vi "EminemStateToNumb.vi"(11 "Eminim_state":T1) -> (3 "StateNumber":dbl)   [LabVIEW 2023]
uses:
  EminemStatesEnum.ctl
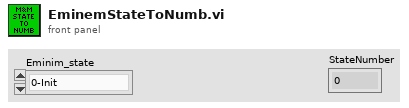
[diagram p1: front panel]
types:
  T1 = typedef "EminemStatesEnum.ctl" = enum16{"0-Init", "1-WaitForCmd", "2-Cancel", "3-ShootStart", "4-ShootRev", "5-ShootUpToSpd?", "6-ShootStartFeed&Timer", "7-ShootTimerOrSensorDone", "8-ShootDone", "9-AmpStart", "10-AmpUpToSpd?", "11-AmpStartFeed&Timer", "12-AmpTimerOrSensorDone", "13-AmpDone"}
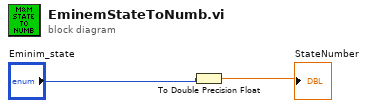
[diagram p0: block diagram]
diagram:
  n1 = To Double Precision Float(number="Eminim_state") -> (double precision float=→"StateNumber":dbl)
